vi "Get Data.vi"(8 "error in":errorcluster, 11 "TE Cooler in":refnum<class "TE Cooler.lvclass">) -> (0 "error out":errorcluster, 2 "Data Out":refnum<class "Data.lvclass">, 3 "TE Cooler out":refnum<class "TE Cooler.lvclass">)   [LabVIEW 2018, in "TE Cooler.lvlib" / "TE Cooler.lvclass"]
doc: "Read the temperature (Input1) off of the controller)."
uses:
  TE Cooler.lvclass
  C:/Users/Labview/Documents/exscalabar_server/Devices/Configurable Device/Configurable Device.lvclass
  reusable/Data/Data.lvclass
  Data/TECData.lvclass
  C:/Users/Labview/Documents/exscalabar_server/reusable/Data/Data.lvclass
  Configurable Device/Configurable Device.lvclass/Configurable Device.ctl
  Data/TECData.lvclass/TECData.ctl
  reusable/Data/Data.lvclass/Data.ctl
  Configurable Device/Read ID.vi
  Data/Data Access/Write Input 1.vi
  Data/Data Access/Write Input 2.vi
  Data/Data Access/Write Power.vi
  reusable/Data/Write Data ID.vi
  reusable/Data/Write measTime.vi
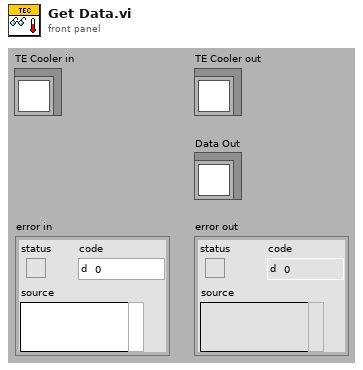
[diagram p1: front panel]
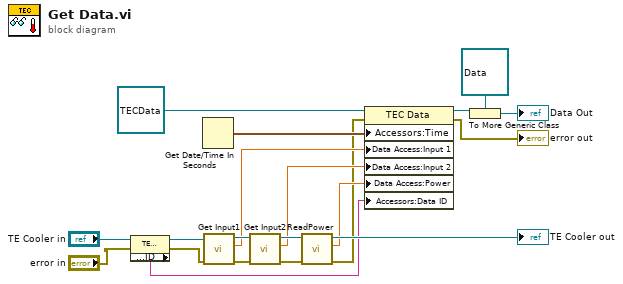
[diagram p0: block diagram]
diagram:
  n1 = property class="TE Tech"(reference="TE Cooler in", error in="error in") -> (reference out=w2:refnum<class "TE Cooler.lvclass">, error out=w3:errorcluster, "Accessors:ID"=w1:string)
  n2 = Get Date/Time In Seconds() -> (seconds since 1Jan1904=w9:timestamp)
  n3 = call "Get Input1.vi"("error in"=w3, "TE Cooler in"=w2) -> ("error out"=w19:errorcluster, "T1"=w10:sgl, "TE Cooler out"=w18:refnum<class "TE Cooler.lvclass">)  [unwired: 7 in]
  n4 = call "Get Input2.vi"("error in"=w19, "TE Cooler in"=w18) -> ("error out"=w15:errorcluster, "T2"=w12:sgl, "TE Cooler out"=w17:refnum<class "TE Cooler.lvclass">)  [unwired: 7 in]
  n5 = call "ReadPower.vi"("error in"=w15, "TE Cooler in"=w17) -> ("error out"=w8:errorcluster, "Power (%)"=w11:sgl, "TE Cooler out"=→"TE Cooler out":refnum<class "TE Cooler.lvclass">)  [unwired: 7 in]
  n6 = property class="TEC Data"(reference=refnum<class "TECData.lvclass"> refnum ("TECData.lvclass"), error in=w8, "Accessors:Time"=w9, "Data Access:Input 1"=w10, "Data Access:Input 2"=w12, "Data Access:Power"=w11, "Accessors:Data ID"=w1) -> (reference out=w13:refnum<class "TECData.lvclass">, error out=→"error out":errorcluster)
  n7 = To More Generic Class(target class=refnum<class "Data.lvclass"> refnum ("Data out"), reference=w13) -> (generic class reference=→"Data Out":refnum<class "Data.lvclass">)
